vi "example.vi"() -> ()   [LabVIEW 2014, in "Que lib.lvlib"]
uses:
  Que lib.lvlib
  Initialise.vi
  Read.vi
  Write.vi
panel:
  out "Recieved data":dbl
  in  "OK Button":bool
  in  "stop":bool
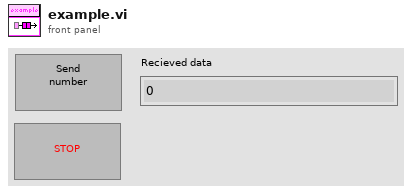
[diagram p1: front panel]
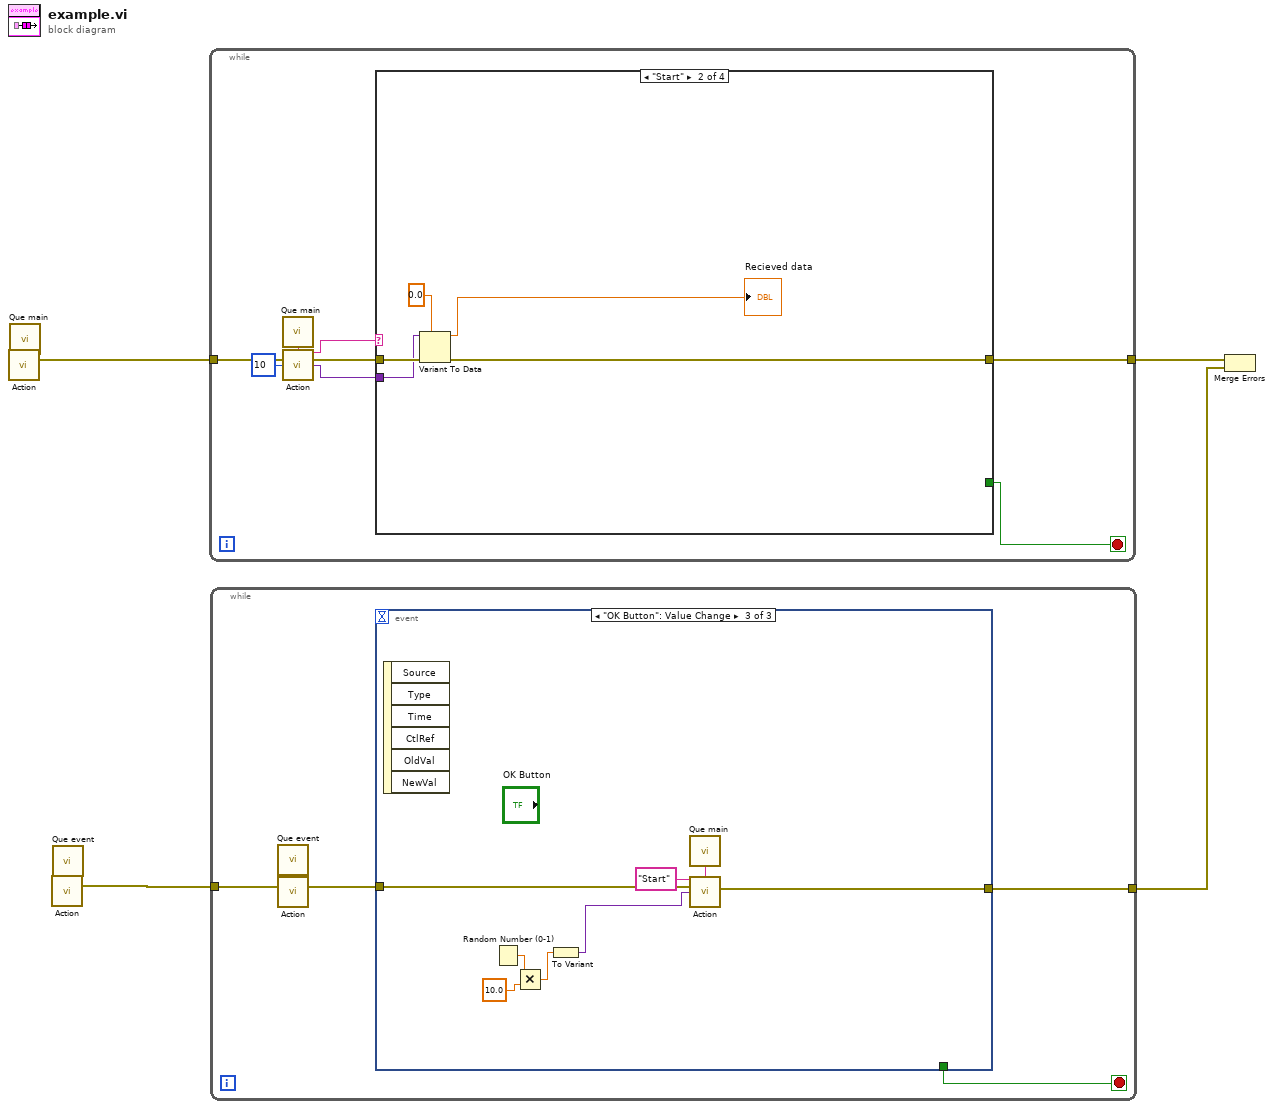
[diagram p0: block diagram]
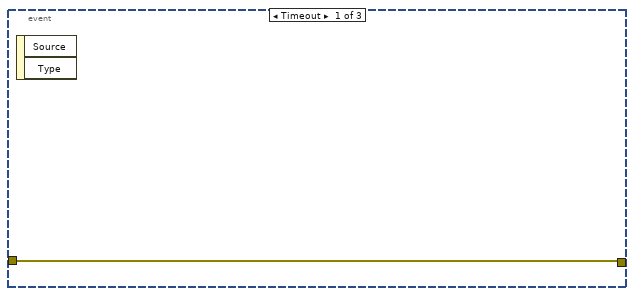
[diagram p2: hidden frame]
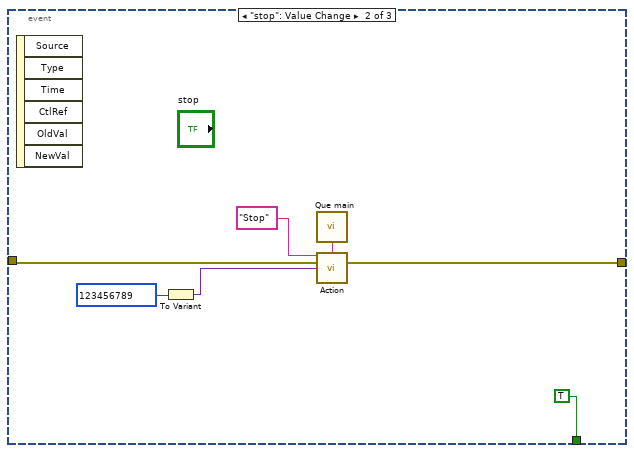
[diagram p3: hidden frame]
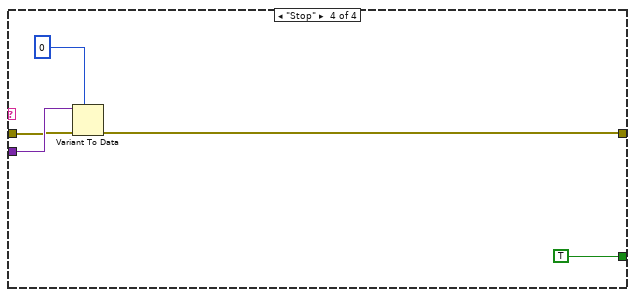
[diagram p6: hidden frame]
diagram:
  n1 = call "Que main.vi"() -> ("Que name"=w6:string)  [unwired: 15 in]
  n2 = call-poly "Action.vi"("Que name"=w6) -> ("error out"=w5:errorcluster)  [unwired: 14 in]
  n3 = call "Que event.vi"() -> ("Que name"=w3:string)  [unwired: 15 in]
  n4 = call-poly "Action.vi"("Que name"=w3) -> ("error out"=w4:errorcluster)  [unwired: 14 in]
  n5 = while {
    tunnel: w5 -> [w14]
    tunnel: [w10] -> w1
    stop <- w9 stop-if-true
    n6 = call "Que main.vi"() -> ("Que name"=w12:string)  [unwired: 15 in]
    n7 = call-poly "Action.vi"("Que name"=w12, "error in"=w14, "Timeout (default 2s)"=10) -> ("Message out"=w11:string, "error out"=w13:errorcluster, "Data"=w7:variant)  [unwired: 10 in]
    n8 = case shown="\"Start\"" w11 {
      tunnel: w13 -> [w15 w20 w21 w24]
      tunnel: [w15 w17 w21 w22] -> w10
      tunnel: [_ _ _ TRUE] -> w9
      tunnel: w7 -> [_ w19 _ w25]
      frame "Initialise" {
      }
      frame "Start" {
        n9 = Variant To Data(error in=w20, type=0.0 ("number (0 to 1)"), Variant=w19) -> (data=→"Recieved data":dbl, error out=w17:errorcluster)
      }
      frame "Run", Default {
      }
      frame "Stop" {
        n10 = Variant To Data(error in=w24, type=0, Variant=w25) -> (error out=w22:errorcluster)  [unwired: 1 out]
      }
    }
  }
  n11 = while {
    tunnel: w4 -> [w31]
    tunnel: [w28] -> w2
    stop <- w27 stop-if-true
    n12 = call "Que event.vi"() -> ("Que name"=w29:string)  [unwired: 15 in]
    n13 = call-poly "Action.vi"("Que name"=w29, "error in"=w31) -> ("error out"=w30:errorcluster)  [unwired: 11 in, 2 out]
    n14 = event shown="[2] \"OK Button\": Value Change" {
      selector: _ -> [_ _ _]
      dyn-events: _ -> [_ _ _]
      timeout: _ -> [_ _ _]
      tunnel: w30 -> [w32 w37 w47]
      tunnel: [w32 w36 w44] -> w28
      tunnel: [_ TRUE _] -> w27
      event Timeout {
        n15 = event-data() -> ()  [unwired: 1 in, 2 out]
      }
      event "stop": Value Change {
        n16 = event-data() -> ()  [unwired: 1 in, 6 out]
        n17 = To Variant(anything=123456789) -> (Variant=w33:variant)
        n18 = call "Que main.vi"() -> ("Que name"=w39:string)  [unwired: 15 in]
        n19 = call-poly "Action.vi"("Message"="Stop" ("Command"), "Que name"=w39, "error in"=w37, "Data"=w33) -> ("error out"=w36:errorcluster)  [unwired: 11 in]
      }
      event "OK Button": Value Change {
        n20 = event-data() -> ()  [unwired: 1 in, 6 out]
        n21 = Random Number (0-1)() -> (number: 0 to 1=w41:dbl)
        n22 = Multiply(x=w41, y=10.0 ("number (0 to 1)")) -> (x*y=w40:dbl)
        n23 = To Variant(anything=w40) -> (Variant=w43:variant)
        n24 = call "Que main.vi"() -> ("Que name"=w46:string)  [unwired: 15 in]
        n25 = call-poly "Action.vi"("Message"="Start" ("Command"), "Que name"=w46, "error in"=w47, "Data"=w43) -> ("error out"=w44:errorcluster)  [unwired: 11 in]
      }
    }
  }
  n26 = Merge Errors(w1, w2) -> ()  [unwired: 1 out]
